vi "CaLabPut.vi"   [LabVIEW 2018]
doc: "This is a polymorphic VI for setting values of EPICS variables.\n\nINPUT:\n <b>PV name(s)</b>\n name of EPICS variable\n Attention: Mixed target data types arise as a result of a 2-D array of size\n (number of names) * (size of largest data type)!\n <b>value(s)</b>\n Boolean value OR Double value OR Double array OR String array\n <b>timeout</b>\n optional\n timeout for Channel Access requests\n <b>error in</b>\n <b>buffer size (since version 1.3 without function)</b>\n <b>synchronous</b>\n optional\n TRUE=synchronous; FALSE=asynchronous\n synchronous = writes value(s) after waiting for end of record processing\n <b>valueSetsInColumns</b>\n optional\n TRUE = use columns for value sets instead of rows\n\nOUTPUT:\n <b>PV name(s)</b>\n name of EPICS variable\n </b>status</b>\n FALSE: request successful\n TRUE: warnings or errors\n <b>errors</b>\n resulting errors of all put commands\n <b>error out</b>\n global io error"
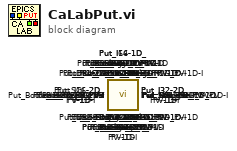
[diagram p0: block diagram]
diagram:
  n1 = call <userlib>:"Put_String-2D_PV-1D-I.vi"() -> ()  [unwired: 8 in, 4 out]
  n2 = call <userlib>:"Put_I32-1D_PV-1D.vi"() -> ()  [unwired: 8 in, 4 out]
  n3 = call <userlib>:"Put_I32-1D_PV.vi"() -> ()  [unwired: 8 in, 4 out]
  n4 = call <userlib>:"Put_Boolean-1D_PV.vi"() -> ()  [unwired: 8 in, 4 out]
  n5 = call <userlib>:"Put_Boolean-1D_PV-I.vi"() -> ()  [unwired: 8 in, 4 out]
  n6 = call <userlib>:"Put_I64-2D_PV-1D-I.vi"() -> ()  [unwired: 8 in, 4 out]
  n7 = call <userlib>:"Put_I64-1D_PV-1D-I.vi"() -> ()  [unwired: 8 in, 4 out]
  n8 = call <userlib>:"Put_I32-1D_PV-I.vi"() -> ()  [unwired: 8 in, 4 out]
  n9 = call <userlib>:"Put_I64_PV-I.vi"() -> ()  [unwired: 8 in, 4 out]
  n10 = call <userlib>:"Put_I32-2D_PV-1D-I.vi"() -> ()  [unwired: 8 in, 4 out]
  n11 = call <userlib>:"Put_I32-1D_PV-1D-I.vi"() -> ()  [unwired: 8 in, 4 out]
  n12 = call <userlib>:"Put_I64-1D_PV-I.vi"() -> ()  [unwired: 8 in, 4 out]
  n13 = call <userlib>:"Put_I32_PV-I.vi"() -> ()  [unwired: 8 in, 4 out]
  n14 = call <userlib>:"Put_I16-2D_PV-1D-I.vi"() -> ()  [unwired: 8 in, 4 out]
  n15 = call <userlib>:"Put_I16-1D_PV-1D-I.vi"() -> ()  [unwired: 8 in, 4 out]
  n16 = call <userlib>:"Put_I16-1D_PV-I.vi"() -> ()  [unwired: 8 in, 4 out]
  n17 = call <userlib>:"Put_I16_PV-I.vi"() -> ()  [unwired: 8 in, 4 out]
  n18 = call <userlib>:"Put_I8-2D_PV-1D-I.vi"() -> ()  [unwired: 8 in, 4 out]
  n19 = call <userlib>:"Put_I8-1D_PV-1D-I.vi"() -> ()  [unwired: 8 in, 4 out]
  n20 = call <userlib>:"Put_I8-1D_PV-I.vi"() -> ()  [unwired: 8 in, 4 out]
  n21 = call <userlib>:"Put_I8_PV-I.vi"() -> ()  [unwired: 8 in, 4 out]
  n22 = call <userlib>:"Put_String-1D_PV-1D-I.vi"() -> ()  [unwired: 8 in, 4 out]
  n23 = call <userlib>:"Put_String-1D_PV-I.vi"() -> ()  [unwired: 8 in, 4 out]
  n24 = call <userlib>:"Put_String_PV-I.vi"() -> ()  [unwired: 8 in, 4 out]
  n25 = call <userlib>:"Put_SGL-2D_PV-1D-I.vi"() -> ()  [unwired: 8 in, 4 out]
  n26 = call <userlib>:"Put_SGL-1D_PV-1D-I.vi"() -> ()  [unwired: 8 in, 4 out]
  n27 = call <userlib>:"Put_SGL-1D_PV-I.vi"() -> ()  [unwired: 8 in, 4 out]
  n28 = call <userlib>:"Put_SGL_PV-I.vi"() -> ()  [unwired: 8 in, 4 out]
  n29 = call <userlib>:"Put_DBL-2D_PV-1D-I.vi"() -> ()  [unwired: 8 in, 4 out]
  n30 = call <userlib>:"Put_DBL-1D_PV-1D-I.vi"() -> ()  [unwired: 8 in, 4 out]
  n31 = call <userlib>:"Put_DBL-1D_PV-I.vi"() -> ()  [unwired: 8 in, 4 out]
  n32 = call <userlib>:"Put_DBL_PV-I.vi"() -> ()  [unwired: 8 in, 4 out]
  n33 = call <userlib>:"Put_Boolean-2D_PV-1D-I.vi"() -> ()  [unwired: 8 in, 4 out]
  n34 = call <userlib>:"Put_Boolean-1D_PV-1D-I.vi"() -> ()  [unwired: 8 in, 4 out]
  n35 = call <userlib>:"Put_SGL-1D_PV.vi"() -> ()  [unwired: 8 in, 4 out]
  n36 = call <userlib>:"Put_I64-1D_PV.vi"() -> ()  [unwired: 8 in, 4 out]
  n37 = call <userlib>:"Put_I16-1D_PV.vi"() -> ()  [unwired: 8 in, 4 out]
  n38 = call <userlib>:"Put_I8-1D_PV.vi"() -> ()  [unwired: 8 in, 4 out]
  n39 = call <userlib>:"Put_DBL-1D_PV.vi"() -> ()  [unwired: 8 in, 4 out]
  n40 = call <userlib>:"Put_String-1D_PV.vi"() -> ()  [unwired: 8 in, 4 out]
  n41 = call <userlib>:"Put_Boolean_PV-I.vi"() -> ()  [unwired: 8 in, 4 out]
  n42 = call <userlib>:"Put_Boolean_PV.vi"() -> ()  [unwired: 8 in, 4 out]
  n43 = call <userlib>:"Put_String-2D_PV-1D.vi"() -> ()  [unwired: 8 in, 4 out]
  n44 = call <userlib>:"Put_String-1D_PV-1D.vi"() -> ()  [unwired: 8 in, 4 out]
  n45 = call <userlib>:"Put_String_PV.vi"() -> ()  [unwired: 8 in, 4 out]
  n46 = call <userlib>:"Put_SGL-2D_PV-1D.vi"() -> ()  [unwired: 8 in, 4 out]
  n47 = call <userlib>:"Put_SGL-1D_PV-1D.vi"() -> ()  [unwired: 8 in, 4 out]
  n48 = call <userlib>:"Put_SGL_PV.vi"() -> ()  [unwired: 8 in, 4 out]
  n49 = call <userlib>:"Put_I64-2D_PV-1D.vi"() -> ()  [unwired: 8 in, 4 out]
  n50 = call <userlib>:"Put_I64-1D_PV-1D.vi"() -> ()  [unwired: 8 in, 4 out]
  n51 = call <userlib>:"Put_I64_PV.vi"() -> ()  [unwired: 8 in, 4 out]
  n52 = call <userlib>:"Put_I32-2D_PV-1D.vi"() -> ()  [unwired: 8 in, 4 out]
  n53 = call <userlib>:"Put_I32_PV.vi"() -> ()  [unwired: 8 in, 4 out]
  n54 = call <userlib>:"Put_I16-2D_PV-1D.vi"() -> ()  [unwired: 8 in, 4 out]
  n55 = call <userlib>:"Put_I16-1D_PV-1D.vi"() -> ()  [unwired: 8 in, 4 out]
  n56 = call <userlib>:"Put_I16_PV.vi"() -> ()  [unwired: 8 in, 4 out]
  n57 = call <userlib>:"Put_I8-2D_PV-1D.vi"() -> ()  [unwired: 8 in, 4 out]
  n58 = call <userlib>:"Put_I8-1D_PV-1D.vi"() -> ()  [unwired: 8 in, 4 out]
  n59 = call <userlib>:"Put_I8_PV.vi"() -> ()  [unwired: 8 in, 4 out]
  n60 = call <userlib>:"Put_DBL-2D_PV-1D.vi"() -> ()  [unwired: 8 in, 4 out]
  n61 = call <userlib>:"Put_DBL-1D_PV-1D.vi"() -> ()  [unwired: 8 in, 4 out]
  n62 = call <userlib>:"Put_DBL_PV.vi"() -> ()  [unwired: 8 in, 4 out]
  n63 = call <userlib>:"Put_Boolean-2D_PV-1D.vi"() -> ()  [unwired: 8 in, 4 out]
  n64 = call <userlib>:"Put_Boolean-1D_PV-1D.vi"() -> ()  [unwired: 8 in, 4 out]
